vi "Bytes to Bits.vi"(1 "Bytes":u8[](array[numeric])) -> (0 "Bits":bool[](array[boolean]))   [LabVIEW 2020, in "LV Tiff.lvlib"]
uses:
  LV Tiff.lvlib
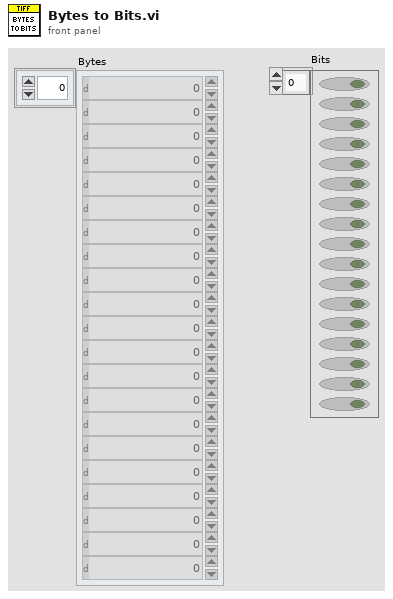
[diagram p1: front panel]
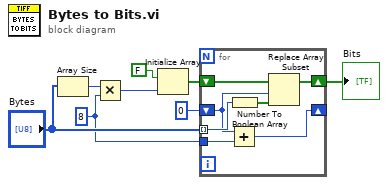
[diagram p0: block diagram]
diagram:
  w1 = 8 ("y")
  n1 = Array Size(array="Bytes") -> (size(s)=w7:i32)
  n2 = Multiply(x=w7, y=w1) -> (x*y=w6:i32)
  n3 = Initialize Array(FALSE, w6) -> (w4:bool[])
  n4 = for {
    tunnel: "Bytes" -> [w15] mode=indexing
    shift-right: [w13] -> w5
    shift-left: w4 -> [w14]
    shift-right: [w11] -> _
    shift-left: 0 ("y") -> [w10]
    tunnel: w1 -> [w9]
    n5 = Add(x=w10, y=w9) -> (x+y=w11:i32)
    n6 = Number To Boolean Array(number=w15) -> (Boolean array=w12:bool[])
    n7 = Replace Array Subset(array=w14, new element=w12, index=w10) -> (w13:bool[])
  }
  "Bits" <- w5
